vi "CreateTrajectory_WriteGlobal_Example.vi"   [LabVIEW 2019]
uses:
  SubVI/StoreTrajectory_GlobalVariable.vi
panel:
  # "Create Trajectory and Write to Global Variable"
  # "See block diagram"
types:
  T1 = typedef "Trajectory_Library.lvlib/TRAJECTORY.ctl" = cluster{"TotalTImeSecs":dbl, "States":T2[]}
  T2 = typedef "Trajectory_Library.lvlib/TRAJ_STATE.ctl" = cluster{"TimeSeconds":dbl, "Velocity":dbl, "Acceleration":dbl, "POSE":T3, "Curvature":dbl}
  T3 = typedef "Trajectory_Library.lvlib/POSE2D.ctl" = cluster{"TRANSLATION":T4, "ROTATION":T5}
  T4 = typedef "Trajectory_Library.lvlib/TRANSLATION2D.ctl" = cluster{"X":dbl, "Y":dbl}
  T5 = typedef "Trajectory_Library.lvlib/ROTATION2D.ctl" = cluster{"VALUE":dbl, "COS":dbl, "SIN":dbl}
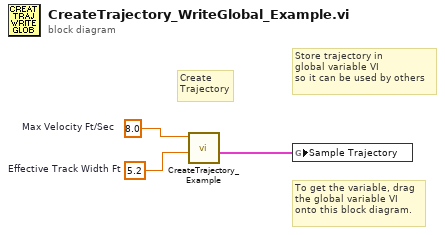
[diagram p0: block diagram]
diagram:
  w2 = 5.2  # Effective Track Width Ft
  w3 = 8.0  # Max Velocity Ft/Sec
  # "To get the variable, drag\nthe global variable VI\nonto this block diagram."
  # "Create\nTrajectory"
  # "Store trajectory in\nglobal variable VI\nso it can be used by others"
  n1 = call "CreateTrajectory_Example.vi"("Effective Track Width Ft"=w2, "Max Velocity Ft/Sec"=w3) -> ("Relative Trajectory"=w1:T1)  [unwired: 6 in, 3 out]
  n2 = global write "StoreTrajectory_GlobalVariable.vi" "Sample Trajectory"(w1) -> ()
